vi "Supervisor.vi"() -> ()   [LabVIEW 2017]
panel:
  out "CTAH Temp In Res Gen":dbl(graph)
  out "Heater Temp Out Res Gen":dbl(graph)
  out "TCHX Temp In Res Gen":dbl(graph)
  out "DHX Temp Out Res Gen":dbl(graph)
  out "CTAH Res Gen":dbl(graph)
  out "Heater Res Gen":dbl(graph)
  in  "Fault Diagnostics Active":bool
  in  "Skip Step":bool
  out "Task Tip":string
  out "Task 3":bool caption="Set pump frequency"
  out "Task 1":bool caption="Reactor Operator"
  out "Task 2":bool caption="Set pump frequency"
  out "Experiment Progress":dbl(slide) max=27.0 scale=0.0..27.0
  in  "error in (no error)":errorcluster
  in  "MATLAB Active":bool
  in  "Stop Supervisor":bool
  in  "Action Recorder ON":bool
  # "Supervisor"
  # "Management Box"
  # "Procedures"
  # "Shared Information"
  # "Information and Action Requests"
  # "NOAH - Networked Operator Analytical Helper"
  # "Fault Information"
  # "Analytics"
  # "Pinned Items"
  # "Grey-Box"
  # "Data-Driven"
  # "Analytical"
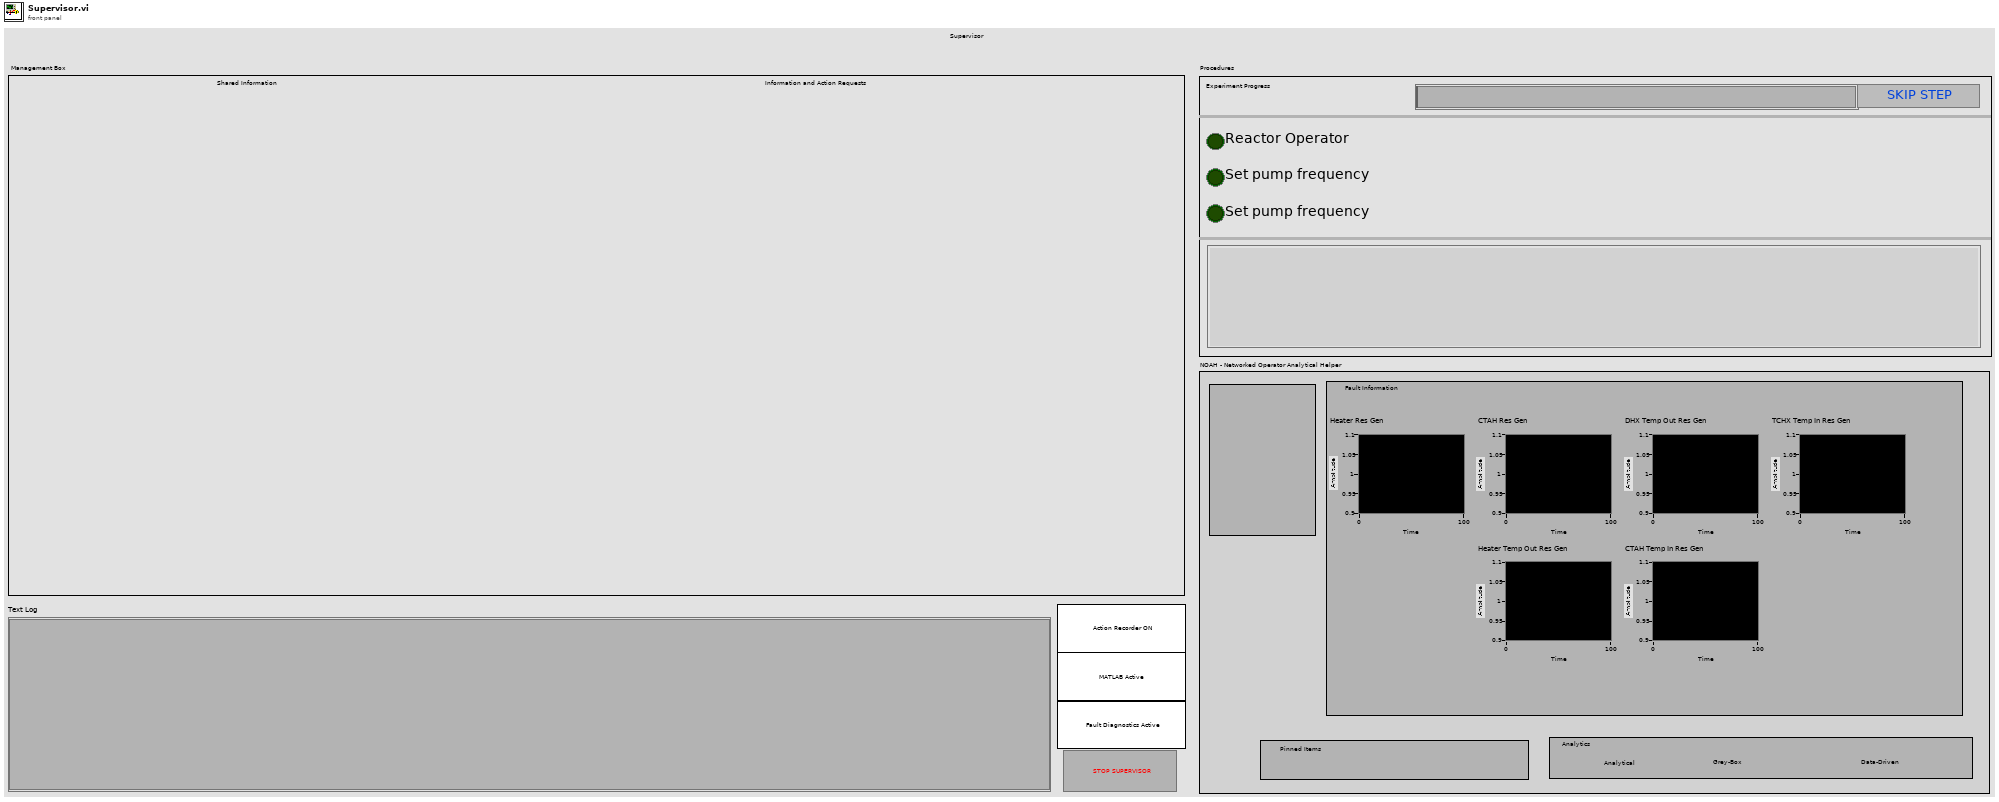
[diagram p1: front panel]
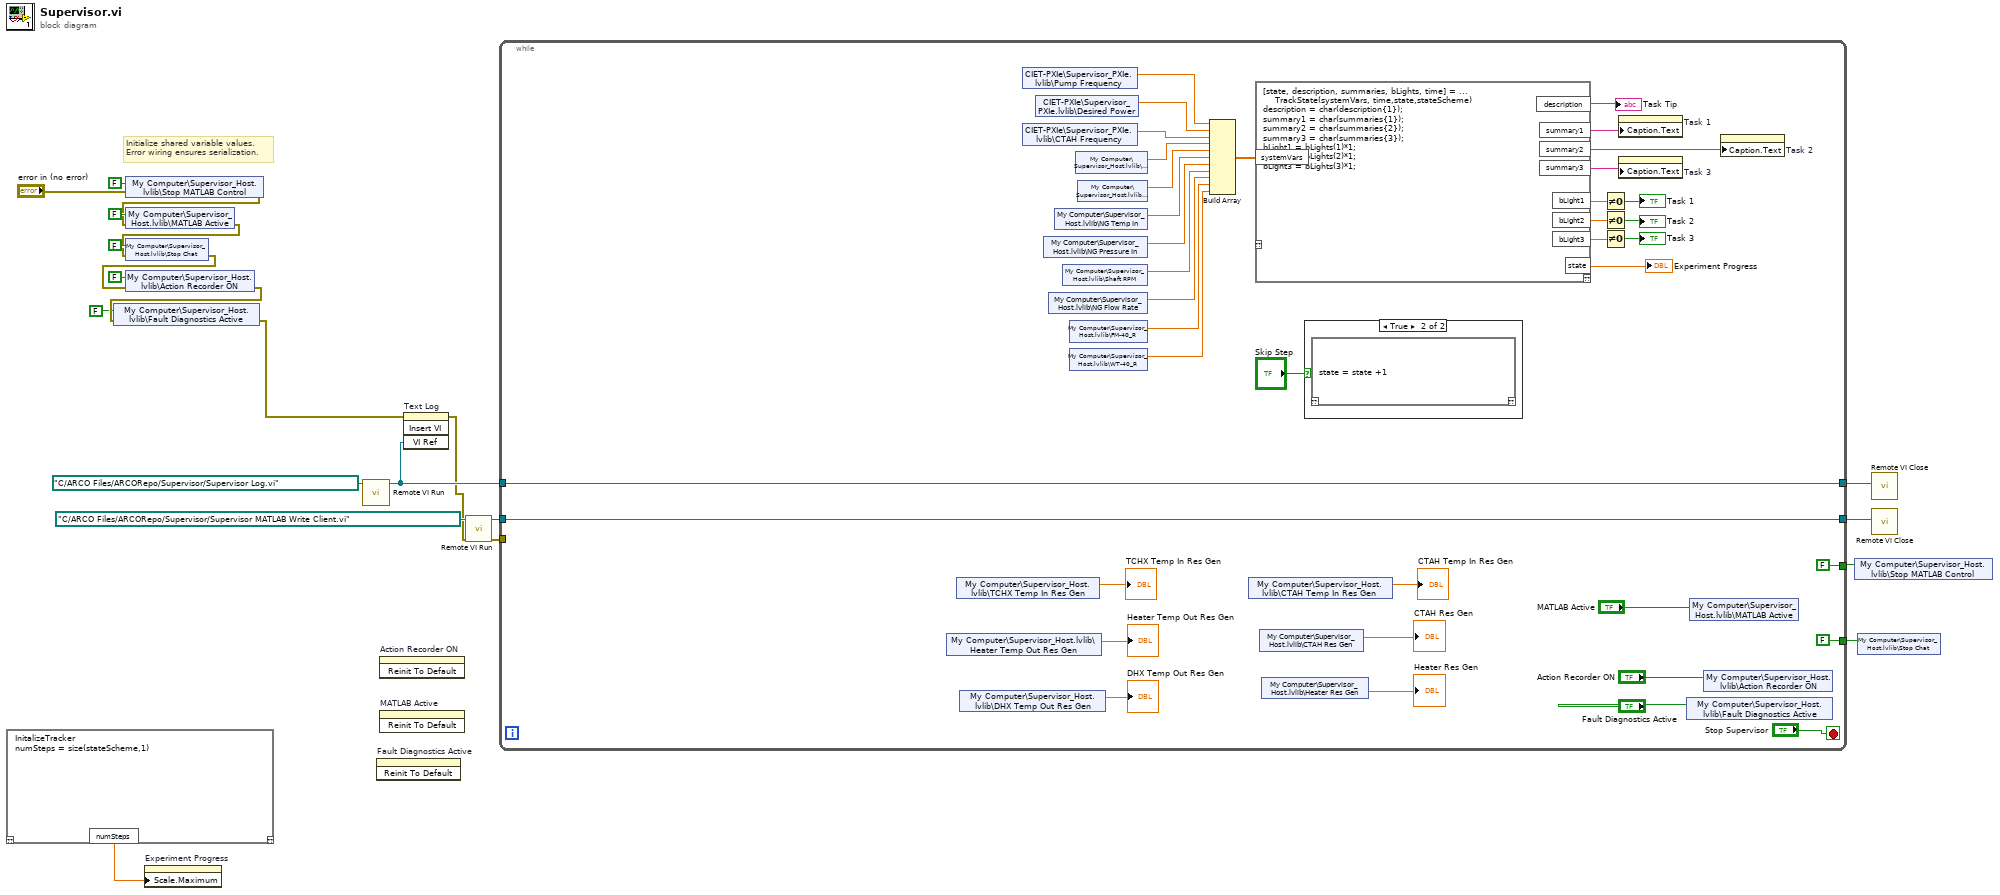
[diagram p0: block diagram]
diagram:
  # "Initialize shared variable values.\nError wiring ensures serialization."
  n1 = script code="InitalizeTracker\nnumSteps = size(stateScheme,1)"() -> ("numSteps"=w6:dbl)  [unwired: 1 in, 1 out]
  n2 = shared-variable "My Computer\\Supervisor_Host.lvlib\\Stop MATLAB Control"(FALSE ("Stop MATLAB Control"), error in="error in (no error)") -> (error out=w10:errorcluster)
  n3 = shared-variable "My Computer\\Supervisor_Host.lvlib\\MATLAB Active"(FALSE ("MATLAB Active"), error in=w10) -> (error out=w9:errorcluster)
  n4 = shared-variable "My Computer\\Supervisor_Host.lvlib\\Stop Chat"(FALSE ("Stop Chat"), error in=w9) -> (error out=w8:errorcluster)
  n5 = shared-variable "My Computer\\Supervisor_Host.lvlib\\Action Recorder ON"(FALSE ("Action Recorder ON"), error in=w8) -> (error out=w2:errorcluster)
  n6 = shared-variable "My Computer\\Supervisor_Host.lvlib\\Fault Diagnostics Active"(FALSE ("Action Recorder ON"), error in=w2) -> (error out=w3:errorcluster)
  n7 = property on="Experiment Progress" class="Slide (strict)"("Scale.Maximum"=w6) -> ()  [unwired: 2 in, 2 out]
  n8 = call "Remote VI Run.vi"("VI Path"=path "C:/ARCO Files/ARCORepo/Supervisor/Supervisor Log.vi") -> ("VI Reference"=w21:refnum<vi>)  [unwired: 9 in, 1 out]
  n9 = invoke on="Fault Diagnostics Active" class="Bool (strict)" method="Reinit To Default"() -> ()  [unwired: 3 in, 3 out]
  n10 = invoke on="Action Recorder ON" class="Bool (strict)" method="Reinit To Default"() -> ()  [unwired: 3 in, 3 out]
  n11 = invoke on="MATLAB Active" class="Bool (strict)" method="Reinit To Default"() -> ()  [unwired: 3 in, 3 out]
  n12 = invoke on="Text Log" class="SubPnl" method="Insert VI"(error in=w3, "VI Ref"=w21) -> (error out=w5:errorcluster)  [unwired: 2 in, 3 out]
  n13 = call "Remote VI Run.vi"("error in (no error)"=w5, "VI Path"=path "C:/ARCO Files/ARCORepo/Supervisor/Supervisor MATLAB Write Client.vi") -> ("error out"=w4:errorcluster, "VI Reference"=w18:refnum<vi>)  [unwired: 8 in]
  n14 = while {
    tunnel: w21 -> [w59]
    tunnel: [w59] -> w20
    tunnel: w18 -> [w56]
    tunnel: [w56] -> w17
    tunnel: [FALSE] -> w16
    tunnel: [FALSE] -> w15
    tunnel: w4 -> [_]
    stop <- "Stop Supervisor" stop-if-true
    n15 = shared-variable "My Computer\\Supervisor_Host.lvlib\\Heater Temp Out Res Gen"() -> (→"Heater Temp Out Res Gen":dbl)  [unwired: 1 in, 1 out]
    n16 = shared-variable "My Computer\\Supervisor_Host.lvlib\\TCHX Temp In Res Gen"() -> (→"TCHX Temp In Res Gen":dbl)  [unwired: 1 in, 1 out]
    n17 = shared-variable "My Computer\\Supervisor_Host.lvlib\\DHX Temp Out Res Gen"() -> (→"DHX Temp Out Res Gen":dbl)  [unwired: 1 in, 1 out]
    n18 = shared-variable "CIET-PXIe\\Supervisor_PXIe.lvlib\\Pump Frequency"() -> (w53:sgl)  [unwired: 1 in, 1 out]
    n19 = shared-variable "CIET-PXIe\\Supervisor_PXIe.lvlib\\CTAH Frequency"() -> (w51:sgl)  [unwired: 1 in, 1 out]
    n20 = shared-variable "CIET-PXIe\\Supervisor_PXIe.lvlib\\Desired Power"() -> (w52:sgl)  [unwired: 1 in, 1 out]
    n21 = shared-variable "My Computer\\Supervisor_Host.lvlib\\NG Pressure In"() -> (w47:sgl)  [unwired: 1 in, 1 out]
    n22 = shared-variable "My Computer\\Supervisor_Host.lvlib\\NG Flow Rate"() -> (w45:sgl)  [unwired: 1 in, 1 out]
    n23 = shared-variable "My Computer\\Supervisor_Host.lvlib\\NG Temp In"() -> (w48:sgl)  [unwired: 1 in, 1 out]
    n24 = shared-variable "My Computer\\Supervisor_Host.lvlib\\Shaft RPM"() -> (w46:sgl)  [unwired: 1 in, 1 out]
    n25 = shared-variable "My Computer\\Supervisor_Host.lvlib\\WT-40_R"() -> (w43:sgl)  [unwired: 1 in, 1 out]
    n26 = shared-variable "My Computer\\Supervisor_Host.lvlib\\FM-40_R"() -> (w44:sgl)  [unwired: 1 in, 1 out]
    n27 = shared-variable "My Computer\\Supervisor_Host.lvlib\\HPT PR"() -> (w50:sgl)  [unwired: 1 in, 1 out]
    n28 = shared-variable "My Computer\\Supervisor_Host.lvlib\\LPT PR"() -> (w49:sgl)  [unwired: 1 in, 1 out]
    n29 = Build Array(w53, w52, w51, w50, w49, w48, w47, w46, w45, w44, w43) -> (w42:sgl[])
    n30 = shared-variable "My Computer\\Supervisor_Host.lvlib\\CTAH Temp In Res Gen"() -> (→"CTAH Temp In Res Gen":dbl)  [unwired: 1 in, 1 out]
    n31 = script code="[state, description, summaries, bLights, time] = ...\n    TrackState(systemVars, time,state,stateScheme)\ndescription = char(description{1});\nsummary1 = char(summaries{1});\nsummary2 = char(summaries{2});\nsummary3 = char(summaries{3});\nbLight1 = bLights(1)*1;\nbLight2 = bLights(2)*1;\nbLight3 = bLights(3)*1;"("systemVars"=w42) -> ("description"=→"Task Tip":string, "summary1"=w30:string, "summary2"=w31:string, "summary3"=w32:string, "bLight1"=w40:dbl, "bLight2"=w39:dbl, "bLight3"=w38:dbl, "state"=→"Experiment Progress":dbl)  [unwired: 1 in, 1 out]
    n32 = shared-variable "My Computer\\Supervisor_Host.lvlib\\CTAH Res Gen"() -> (→"CTAH Res Gen":dbl)  [unwired: 1 in, 1 out]
    n33 = shared-variable "My Computer\\Supervisor_Host.lvlib\\Heater Res Gen"() -> (→"Heater Res Gen":dbl)  [unwired: 1 in, 1 out]
    n34 = case shown="True" "Skip Step" {
      frame False {
      }
      frame True {
        n35 = script code="state = state +1"() -> ()  [unwired: 1 in, 1 out]
      }
    }
    n36 = Not Equal To 0?(x=w40) -> (x != 0?=→"Task 1":bool)
    n37 = Not Equal To 0?(x=w39) -> (x != 0?=→"Task 2":bool)
    n38 = Not Equal To 0?(x=w38) -> (x != 0?=→"Task 3":bool)
    n39 = property on="Task 1" class="Bool (strict)"("Caption.Text"=w30) -> ()  [unwired: 2 in, 2 out]
    n40 = property on="Task 3" class="Bool (strict)"("Caption.Text"=w32) -> ()  [unwired: 2 in, 2 out]
    n41 = shared-variable "My Computer\\Supervisor_Host.lvlib\\Fault Diagnostics Active"("Fault Diagnostics Active") -> ()  [unwired: 1 in, 1 out]
    n42 = shared-variable "My Computer\\Supervisor_Host.lvlib\\MATLAB Active"("MATLAB Active") -> ()  [unwired: 1 in, 1 out]
    n43 = shared-variable "My Computer\\Supervisor_Host.lvlib\\Action Recorder ON"("Action Recorder ON") -> ()  [unwired: 1 in, 1 out]
    n44 = property on="Task 2" class="Bool (strict)"("Caption.Text"=w31) -> ()  [unwired: 2 in, 2 out]
  }
  n45 = shared-variable "My Computer\\Supervisor_Host.lvlib\\Stop MATLAB Control"(w15) -> ()  [unwired: 1 in, 1 out]
  n46 = shared-variable "My Computer\\Supervisor_Host.lvlib\\Stop Chat"(w16) -> ()  [unwired: 1 in, 1 out]
  n47 = call "Remote VI Close.vi"("reference"=w20) -> ()  [unwired: 9 in, 2 out]
  n48 = call "Remote VI Close.vi"("reference"=w17) -> ()  [unwired: 9 in, 2 out]
